vi "DeleteFunction (SubVI).vi"(11 "Protocol":refnum<vi>) -> ()   [LabVIEW 2017]
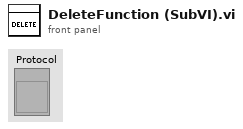
[diagram p1: front panel]
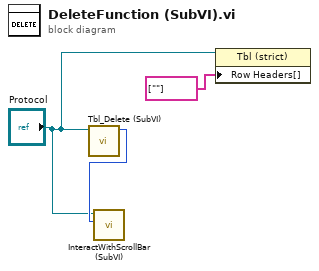
[diagram p0: block diagram]
diagram:
  n1 = call "Tbl_Delete (SubVI).vi"("Table in"="Protocol") -> ("element"=w3:i32)  [unwired: 10 in]
  n2 = call "InteractWithScrollBar (SubVI).vi"("element"=w3, "Table in"="Protocol") -> ()  [unwired: 10 in]
  n3 = property on="Property Node" class="Tbl (strict)"(reference="Protocol", "Row Headers[]"=string[] [""] ("Row Header Strings[]")) -> ()  [unwired: 1 in, 2 out]
